vi "To 1D Path Tree Data.vi"(10 "1D Path":path[](array[path])) -> (3 "1D Path Tree Data":refnum<class "1D Path.lvclass">)   [LabVIEW 2020, in "NI_VIAnCFGDataStructure.lvlib" / "1D Path.lvclass"]
doc: "Convert a 1D Path value to Tree Data type."
uses:
  <vilib>/addons/analyzer/VIAnCFGDataStructure/Data Types/Path Array/1D Path.lvclass
  <vilib>/addons/analyzer/VIAnCFGDataStructure/Data Types/Path Array/1D Path.lvclass/1D Path.ctl
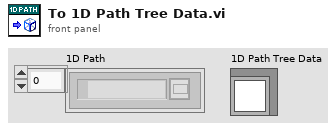
[diagram p1: front panel]
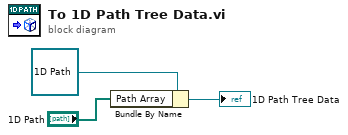
[diagram p0: block diagram]
diagram:
  n1 = Bundle By Name(cluster=refnum<class "1D Path.lvclass"> refnum ("Path Array.lvclass"), "Path Array"="1D Path") -> (→"1D Path Tree Data":refnum<class "1D Path.lvclass">)
